vi "RebootSystem.vi"(8 "error in (no error)":errorcluster) -> (0 "error out":errorcluster)   [LabVIEW 2017, in "SystemInfoProcess.lvlib"]
doc: "Reboots the system on command."
uses:
  <vilib>/addons/SystemInfoProcess/SystemInfoProcess.lvlib
  <vilib>/nisyscfg/nisyscfg.lvlib
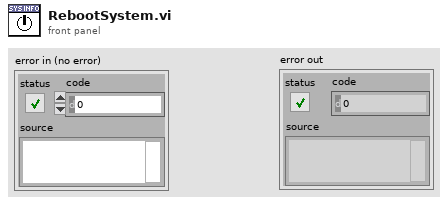
[diagram p1: front panel]
types:
  T1 = enum16{"open", "replace", "create", "open or create", "replace or create", "replace or create with confirmation"}
  T2 = typedef "PointValueMap.lvlib/PointMap.ctl" = refnum<data-value>
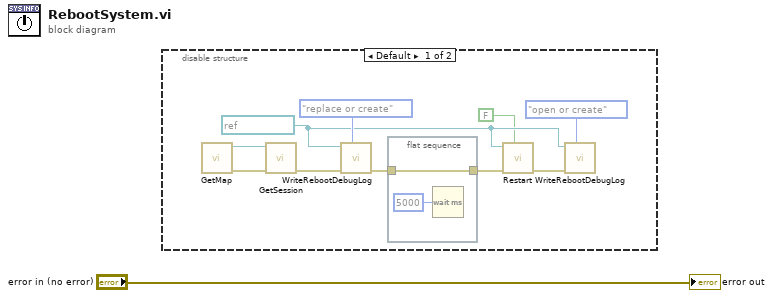
[diagram p0: block diagram]
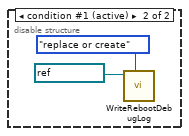
[diagram p2: hidden frame]
diagram:
  n1 = disable-structure shown="Default" {
    frame condition #0 {
      w3 = refnum<k21> "127.0.0.1" ("session")
      n2 = call <vilib>:"GetMap.vi"() -> ("error out"=w11:errorcluster, "SystemInfoMap"=w10:T2)  [unwired: 10 in]
      n3 = call <vilib>:"GetSession.vi"("error in (no error)"=w11, "map"=w10) -> ("error out"=w9:errorcluster)  [unwired: 8 in, 1 out]
      n4 = call <vilib>:"WriteRebootDebugLog.vi"("operation (0:open)"=T1."replace or create", "error in"=w9, "session"=w3) -> ("error out"=w7:errorcluster)  [unwired: 8 in]
      n5 = flat-sequence {
        tunnel: [w13] -> w8
        tunnel: w7 -> [w13]
        frame #0 {
          n6 = Wait (ms)(milliseconds to wait=u32 5000) -> ()  [unwired: 1 out]
        }
      }
      n7 = call <vilib>:"Restart.vi"("Wait Until Complete (T)"=FALSE, "error in (no error)"=w8, "Session in"=w3) -> ("error out"=w5:errorcluster)  [unwired: 6 in, 2 out]
      n8 = call <vilib>:"WriteRebootDebugLog.vi"("operation (0:open)"=T1."open or create", "error in"=w5, "session"=w3) -> ()  [unwired: 8 in, 1 out]
    }
    frame condition #1 (active) {
      n9 = call <vilib>:"WriteRebootDebugLog.vi"("operation (0:open)"=T1."replace or create", "session"=refnum<k21> "desktop") -> ()  [unwired: 9 in, 1 out]
    }
  }
  "error out" <- "error in (no error)"
